vi "Time_stamp.vi"() -> (0 "date/time string":string, 1 "date string":string)   [LabVIEW 2017]
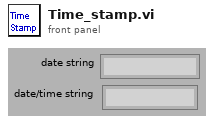
[diagram p1: front panel]
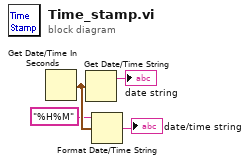
[diagram p0: block diagram]
diagram:
  n1 = Get Date/Time In Seconds() -> (seconds since 1Jan1904=w3:timestamp)
  n2 = Get Date/Time String(seconds (now)=w3) -> (date string=→"date string":string)  [unwired: 3 out]
  n3 = Format Date/Time String(time format string (%c)="%H%M", seconds (now)=w3) -> (date/time string=→"date/time string":string)  [unwired: 1 out]
